vi "Experiment_Control.vi"() -> ()   [LabVIEW 2014]
uses:
  Controls/ExperimentControlEnum.ctl
  Controls/DAQ Channel Array.ctl
  Controls/DAQ Card-Channel Settings.ctl
  Controls/DAQ Card Channel Array.ctl
  Controls/DAQ Channel Settings.ctl
  Controls/DAQ Card Settings.ctl
  Controls/DIOTypedef.ctl
  Controls/TimingControlArray.ctl
  Controls/TimingControl.ctl
  Controls/TimingControlChannel.ctl
  Controls/TimeIncrementCluster.ctl
  Controls/TimingPlot.ctl
  Controls/ExperimentControlCluster.ctl
  Controls/ShotQualityEnum.ctl
panel:
  in  "Exit Program":bool
  in  "Restore Default Settings":bool
  in  "Tab Control":T1(tab)
  out "Program Version":string
  in  "Resume from previous shot":bool
  out "Timing Plot":T2
  in  "Load Shot Settings":bool
  in  "Load a previous shot?":i32
  in  "Shot Quality":enum32{"-2", "-1", "1", "2", "3", "0"}(radio)=enum."0"
  in  "Select MDS+ Data Tree":string(combo)="proto_tree"
  in  "Discard shot data":bool
  in  "Save shot data":bool
  in  "Increments":T3
  in  "Timing Array":T4 {"Timing Sequence"."Dt" format="%_3p"; "Timing Sequence"."Time" format="%_3p"}
  in  "Shot Notes":string
  out "Time":string
  out "System State":T7=enum."FIRE: Trigger"
  in  "Abort":bool
  in  "Fire Experiment":bool
  out "System Message":string
  out "Next Shot #":i32
  in  "DAQ Channel Array":T8 {"Card Settings"."Start Time" format="%#_3p"; "Card Settings"."End Time" format="%#_3p"; "Card Settings"."Rate" format="%#_3p"}
  in  "DIO Cluster":T13
  # "Save the current shot?"
  # "Time [s]"
  # "Channel                                     Name                                                               Voltage Range                    Card Settings"
  # "Sampling Rate [1/s]"
  # "Start Time [s]"
  # "End Time [s]"
  # "On/Off      Channel                     Name"
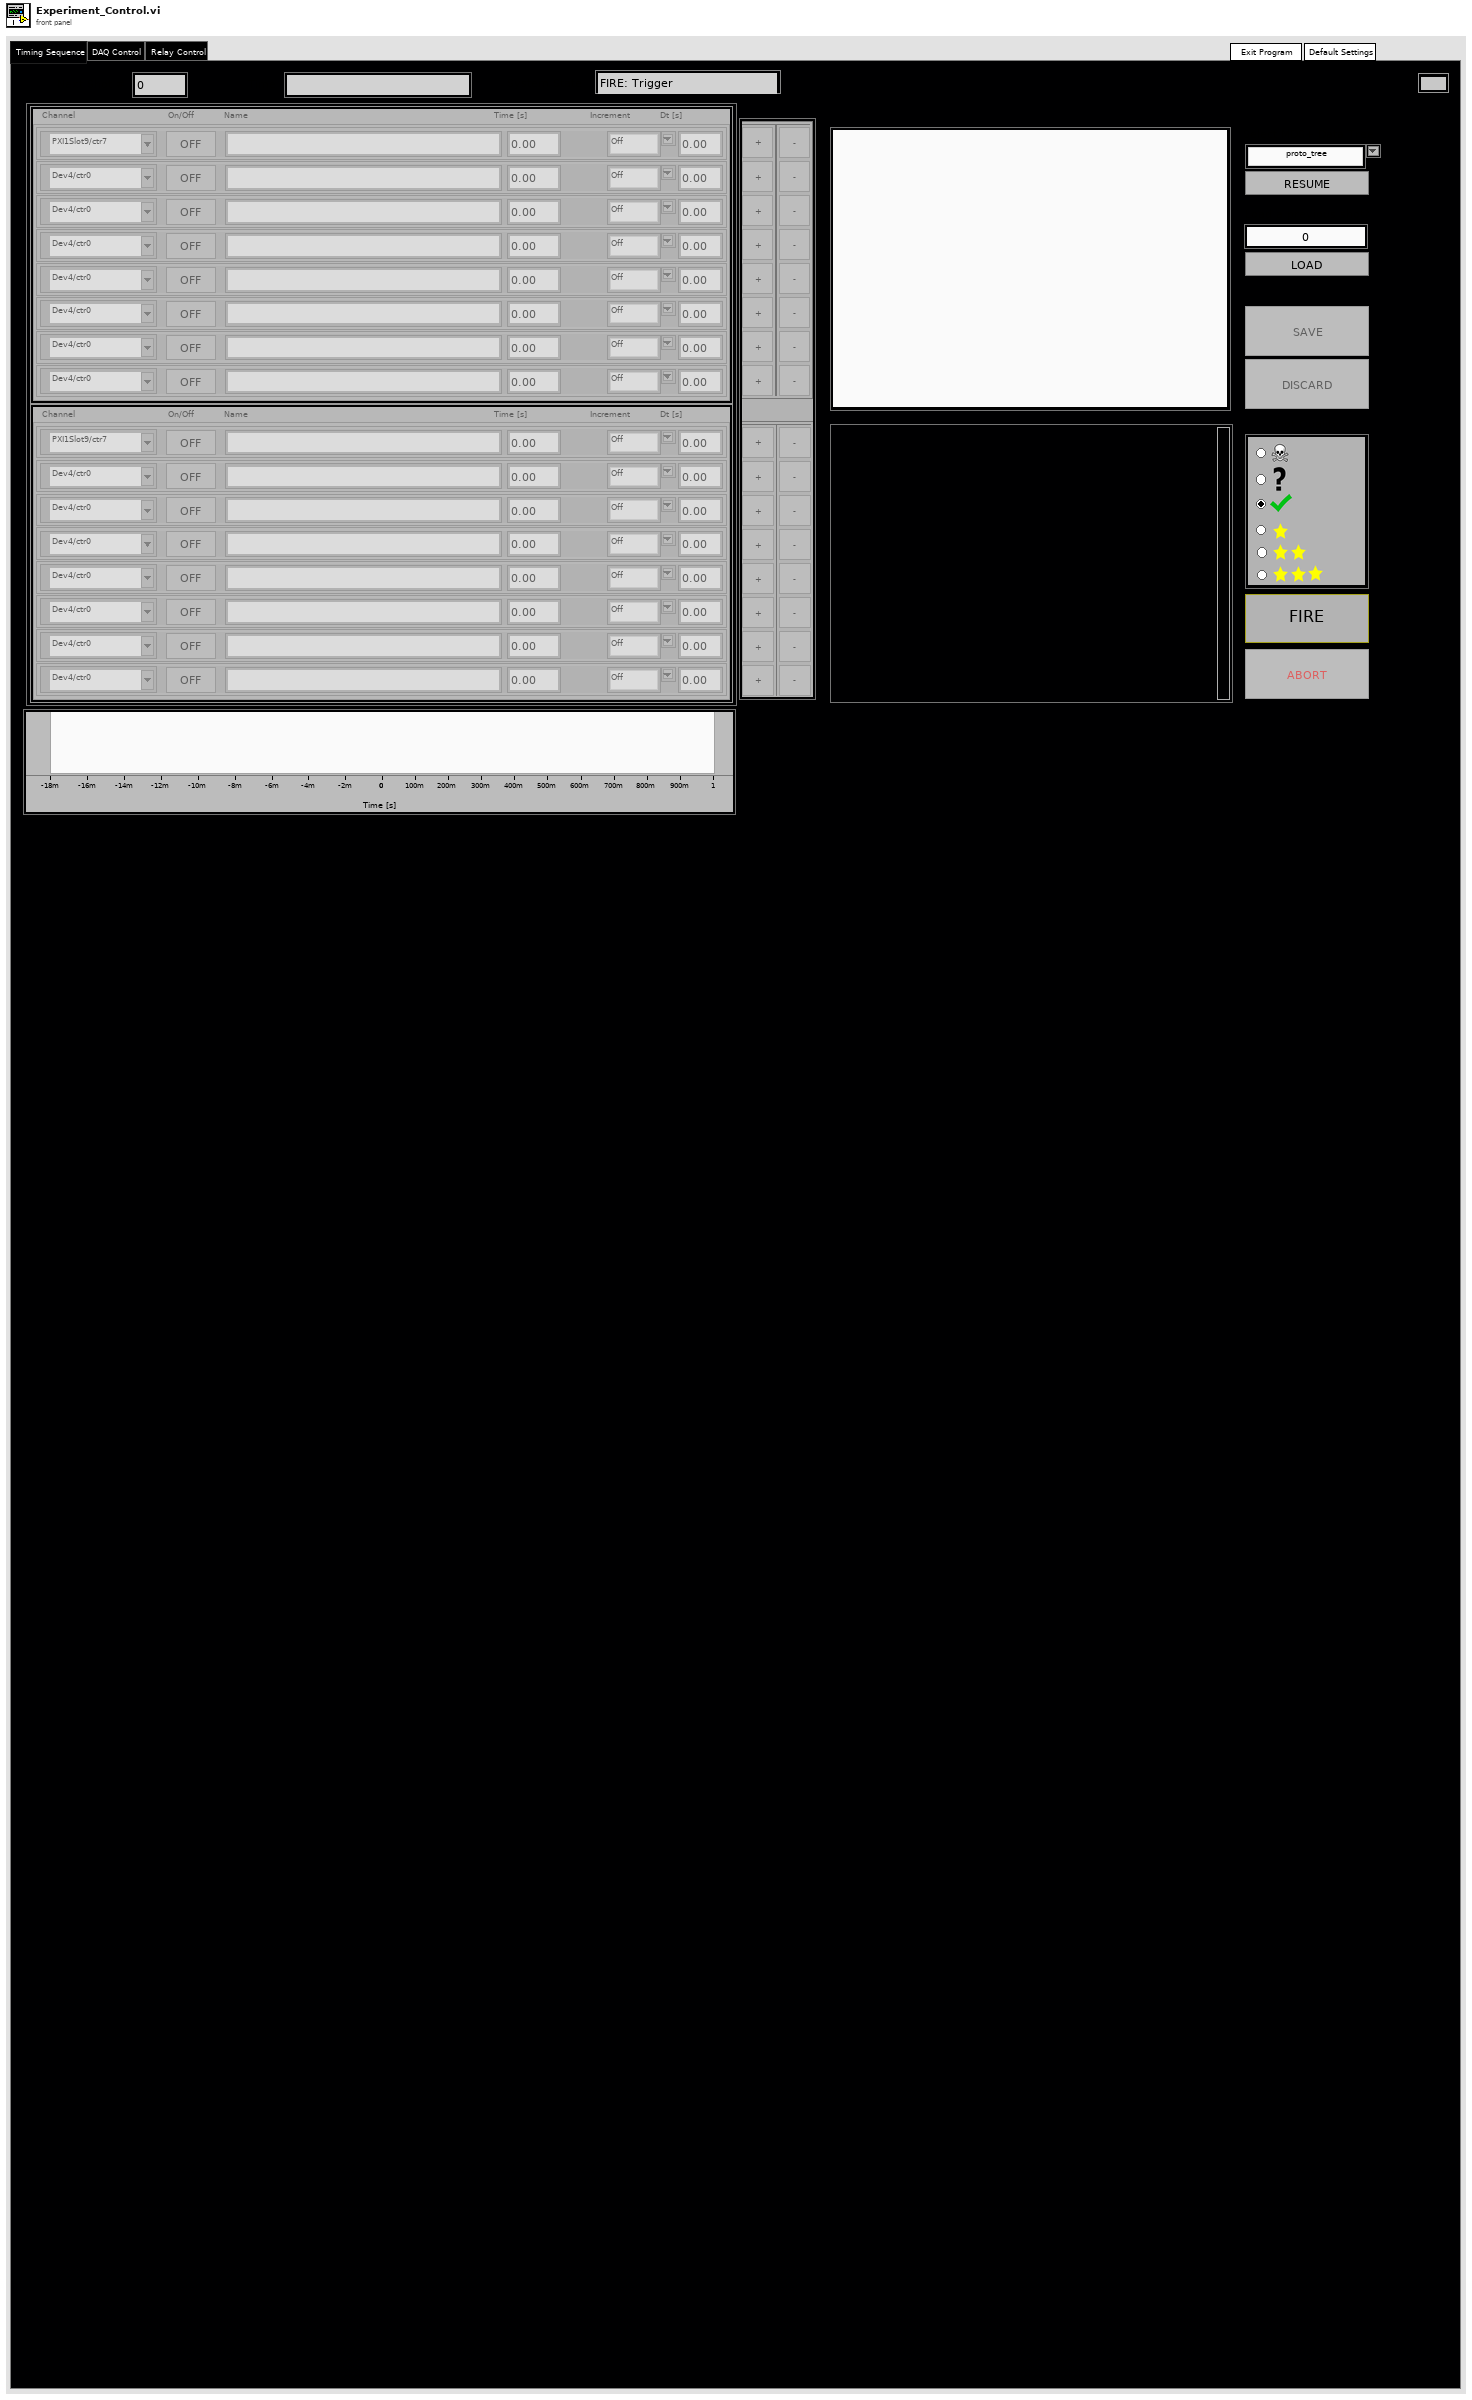
[diagram p1: front panel]
types:
  T1 = enum32{"Timing Sequence", "DAQ Control", "Relay Control"}
  T2 = typedef "TimingPlot.ctl" = cluster{"Negative Time Graph":cluster{dbl[], dbl[]}[], "Positive Time Graph":cluster{dbl[], dbl[]}[], "XY Graph":cluster{"X":dbl[], "Y":dbl[]}[]}
  T3 = typedef "TimeIncrementCluster.ctl" = cluster{"Plus Minus":cluster{"Add 1":cluster{"plus 1":bool, "plus 2":bool, "plus 3":bool, "plus 4":bool, "plus 5":bool, "plus 6":bool, "plus 7":bool, "plus 8":bool}, "Minus 1":cluster{"minus 1":bool, "minus 2":bool, "minus 3":bool, "minus 4":bool, "minus 5":bool, "minus 6":bool, "minus 7":bool, "minus 8":bool}}, "Plus Minus 2":cluster{"Add 1":cluster{"plus 1":bool, "plus 2":bool, "plus 3":bool, "plus 4":bool, "plus 5":bool, "plus 6":bool, "plus 7":bool, "plus 8":bool}, "Minus 1":cluster{"minus 1":bool, "minus 2":bool, "minus 3":bool, "minus 4":bool, "minus 5":bool, "minus 6":bool, "minus 7":bool, "minus 8":bool}}}
  T4 = typedef "TimingControlArray.ctl" = T5[]
  T5 = typedef "TimingControl.ctl" = cluster{"Timing Sequence":T6[]}
  T6 = typedef "TimingControlChannel.ctl" = cluster{"Active":bool, "counter":tag, "Channel Name":string, "Time":dbl, "Increment":string, "Dt":dbl}
  T7 = typedef "ExperimentControlEnum.ctl" = enum16{"Idle", "FIRE: Read Panel Settings", "FIRE: Generate Tasks", "FIRE: Set DAQ Triggers", "FIRE: Trigger", "FIRE: Wait for Task Completion", "FIRE: Read out DAQs", "Write to MDS+", "Clear Tasks", "Stop VI", "DIO Change", "Turn Off DIO", "Update Tree", "Load Shot Settings", "Restore Default Settings"}
  T8 = typedef "DAQ Channel Array.ctl" = T9[]
  T9 = typedef "DAQ Card-Channel Settings.ctl" = cluster{"DAQ Channel Array":T10, "Card Settings":T12}
  T10 = typedef "DAQ Card Channel Array.ctl" = T11[]
  T11 = typedef "DAQ Channel Settings.ctl" = cluster{"Active":bool, "Channel Name":string, "Channel":tag, "Voltage Range":string}
  T12 = typedef "DAQ Card Settings.ctl" = cluster{"Rate":dbl, "End Time":dbl, "Start Time":dbl}
  T13 = typedef "DIOTypedef.ctl" = cluster{"DIO Booleans":bool[], "DIO Channel Array":cluster{"Channel Name":string, "DIO lines":tag}[]}
  T14 = typedef "ExperimentControlCluster.ctl" = cluster{"Experiment Control":T7, "Variant":variant}
  T15 = typedef "ExperimentStateCluster.ctl" = cluster{"error":errorcluster, "Digitizer DAQmx Tasks":cluster{"TaskArray":refnum<k21>[]}, "Digitizer Settings":cluster{"Channel Settings":T16[][], "Card Settings":T17}, "Synchronization Settings":cluster{"Synchronizer":refnum<k15>, "source terminal":string}, "Digitizer Data":waveform(dbl)[][], "Next Shot#":string, "System Message":string, "User Shot Notes":string, "Timing Settings":T19, "Timing Tasks":cluster{"TaskArray":refnum<k21>[][]}, "Tree":string, "Time Card/Channels":i32[], "DAQ Card/Channels":i32[], "Program Version":string}
  T16 = typedef "DigitizerSettingsChannelSettings.ctl" = cluster{"Channel":tag, "Channel Name":string, "Voltage Range":dbl, "Active":bool}
  T17 = typedef "DigitizerSettingsCardSettingsArray.ctl" = T18[]
  T18 = typedef "DigitizerSettingsCardSettings.ctl" = cluster{"Start Time":dbl, "End Time":dbl, "Sample Rate":dbl, " Pre-Trigger Samples":u32, "Total Samples":i32, "Samples to Remove":u32, "Trigger Source":tag, "Global Edge Type":i32, "PXIStarLine":tag}
  T19 = typedef "TimingSettings.ctl" = cluster{"Timing Card Settings":T20[], "Timing Channel Settings":T21[][]}
  T20 = typedef "TimingCardSettings.ctl" = cluster{"Trigger Source":tag, "Clock Source":tag, "PXIStarLine":tag}
  T21 = typedef "TimingChannelSettings.ctl" = cluster{"Delay (s)":dbl, "Pulse width (s)":dbl, "Active":bool, "Channel Name":string, "counter":tag, "FrontPanelTime":dbl}
  T22 = cluster{"DAQ Channel Array":T10, "Card Settings":T12}[]
  T23 = typedef "ShotQualityEnum.ctl" = enum32{"-2", "-1", "1", "2", "3", "0"}
  T24 = cluster{"Channel Name":string, "DIO lines":tag}[]
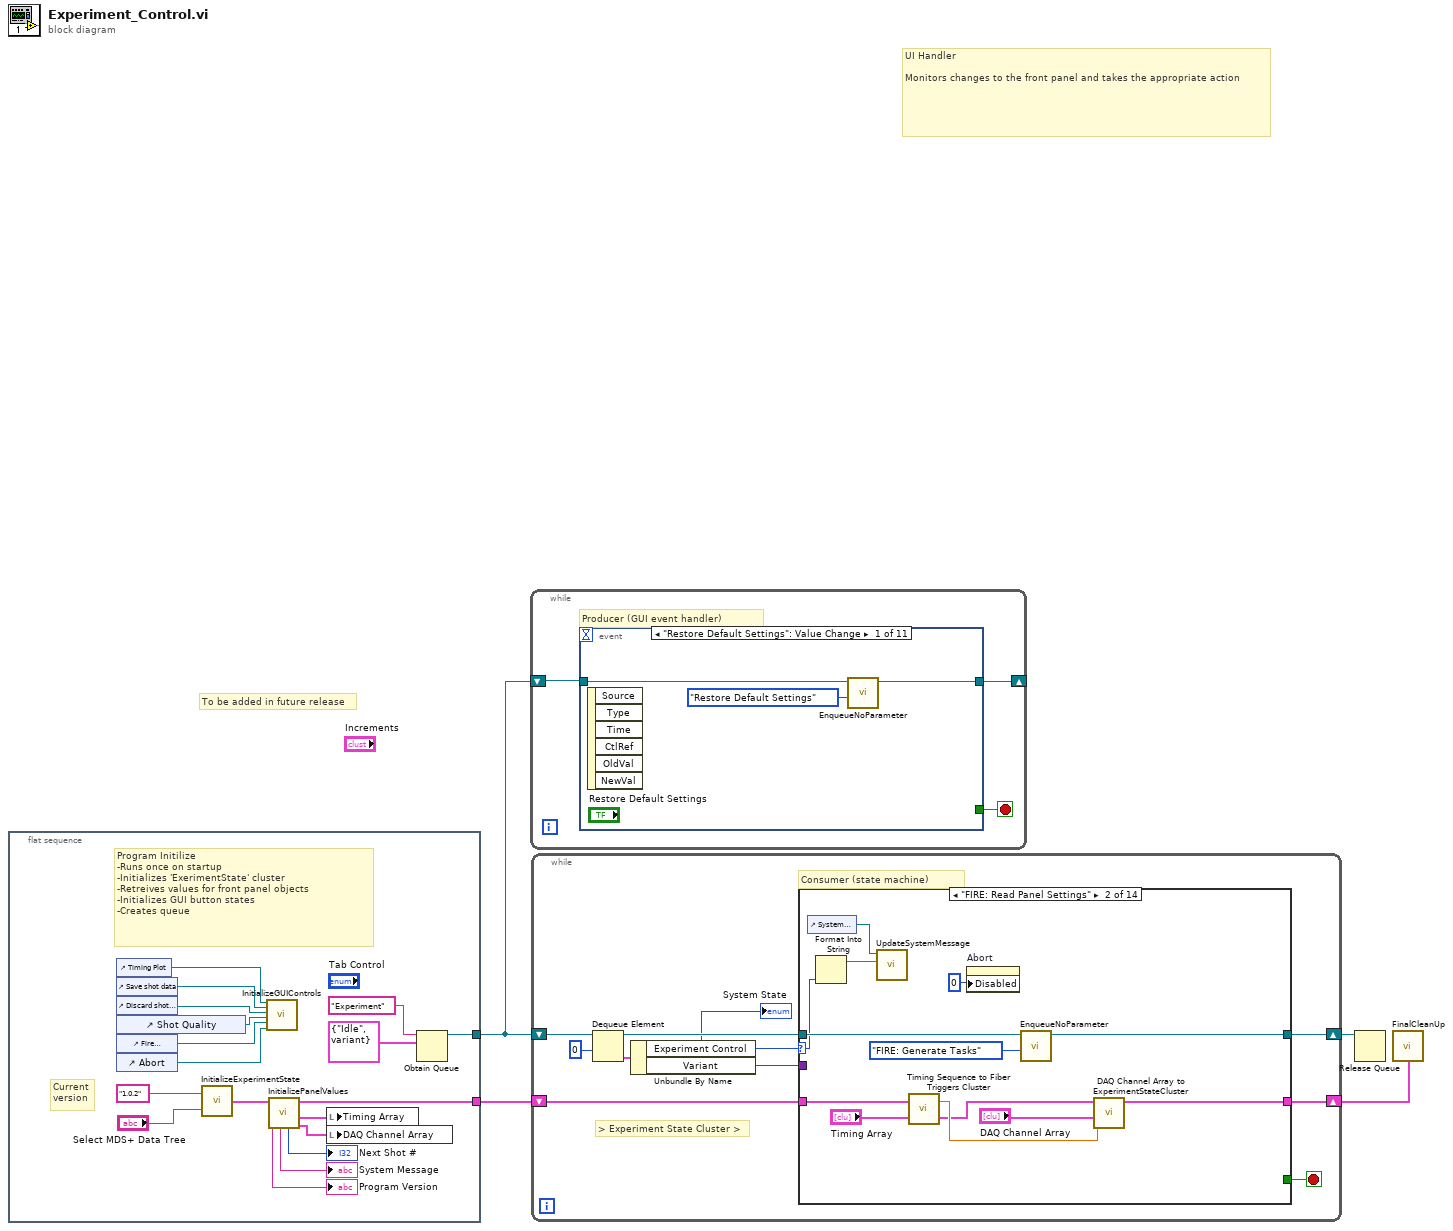
[diagram p0: block diagram]
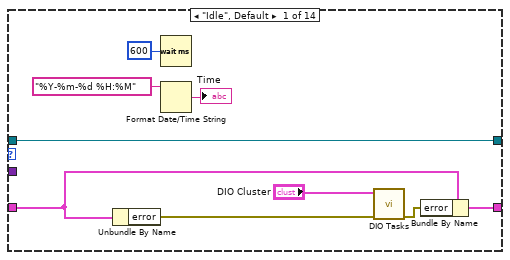
[diagram p2: hidden frame]
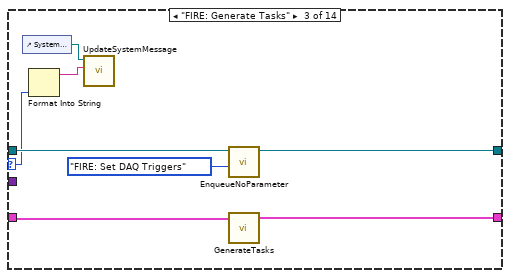
[diagram p3: hidden frame]
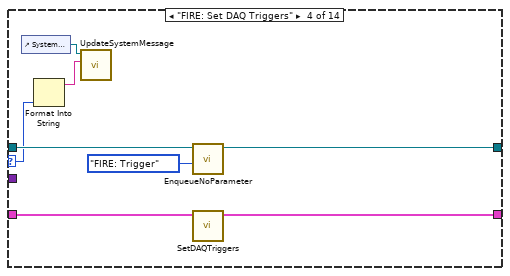
[diagram p4: hidden frame]
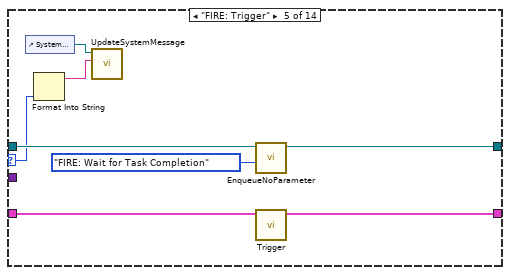
[diagram p5: hidden frame]
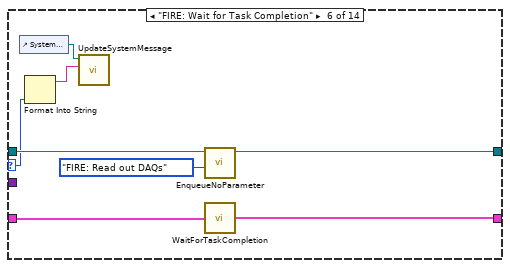
[diagram p6: hidden frame]
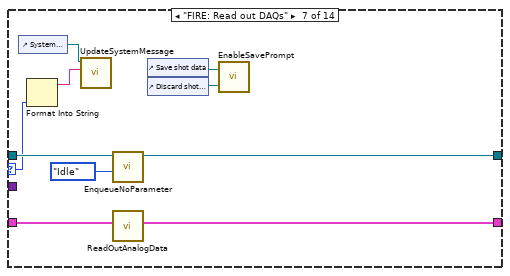
[diagram p7: hidden frame]
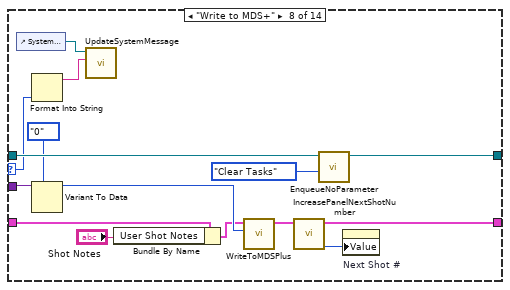
[diagram p8: hidden frame]
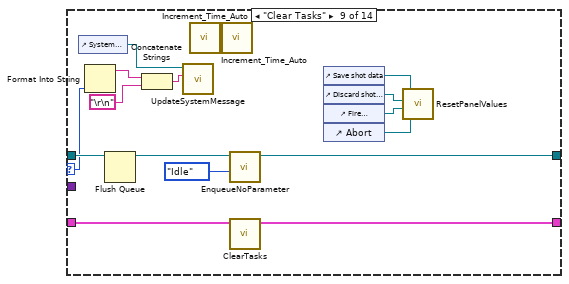
[diagram p9: hidden frame]
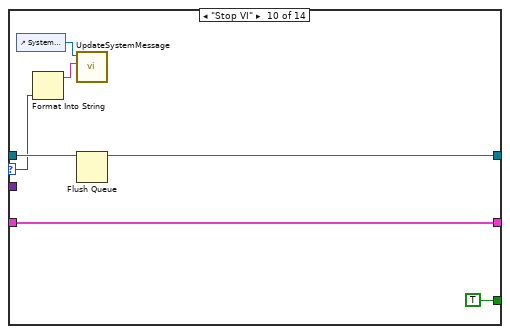
[diagram p10: hidden frame]
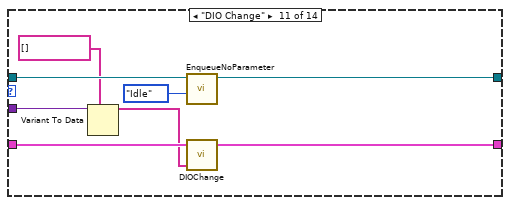
[diagram p11: hidden frame]
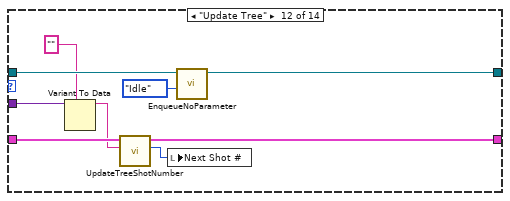
[diagram p12: hidden frame]
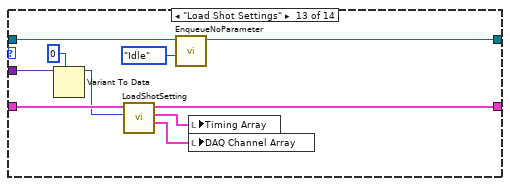
[diagram p13: hidden frame]
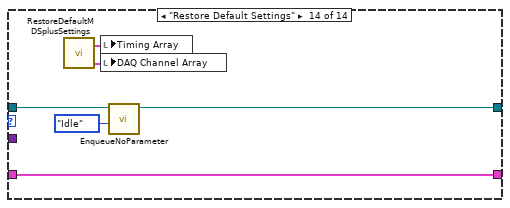
[diagram p14: hidden frame]
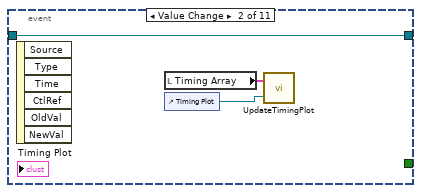
[diagram p15: hidden frame]
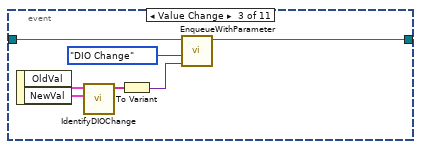
[diagram p16: hidden frame]
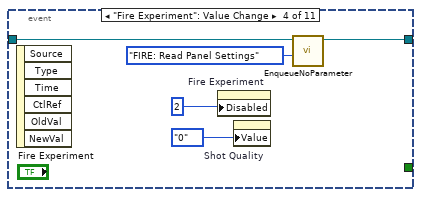
[diagram p17: hidden frame]
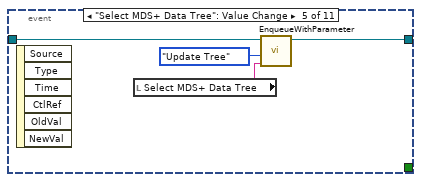
[diagram p18: hidden frame]
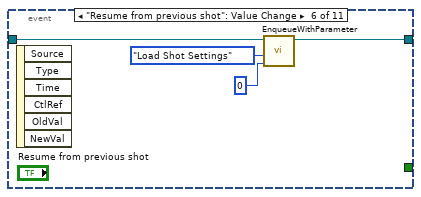
[diagram p19: hidden frame]
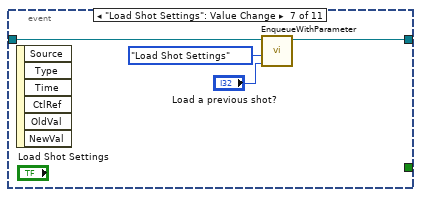
[diagram p20: hidden frame]
diagram:
  # "To be added in future release"
  # "UI Handler\n\nMonitors changes to the front panel and takes the appropriate action"
  n1 = flat-sequence {
    tunnel: [w21] -> w4
    tunnel: [w10] -> w3
    frame #0 {
      # "Current\nversion"
      # "Program Initilize\n-Runs once on startup\n-Initializes 'ExerimentState' cluster\n-Retreives values for front panel objects\n-Initializes GUI button states\n-Creates queue"
      n2 = control-ref of="Timing Plot"() -> (w17:refnum<vi>)
      n3 = control-ref of="Save shot data"() -> (w16:refnum<vi>)
      n4 = control-ref of="Discard shot data"() -> (w15:refnum<vi>)
      n5 = control-ref of="Shot Quality"() -> (w12:refnum<vi>)
      n6 = control-ref of="Fire Experiment"() -> (w13:refnum<vi>)
      n7 = control-ref of="Abort"() -> (w14:refnum<vi>)
      n8 = call "InitializeExperimentState.vi"("Tree Name"="Select MDS+ Data Tree", "Program Version"="1.0.2" ("string")) -> ("Experiment State"=w11:T15)
      n9 = call "InitializeGUIControls.vi"("Timing Plot"=w17, "Save shot data"=w16, "Discard shot data"=w15, "Shot Quality"=w12, "Fire Experiment"=w13, "Abort"=w14) -> ()  [unwired: 14 in]
      n10 = call "InitializePanelValues.vi"("Experiment State in"=w11) -> ("Initialized DAQ Array"=w8:T22, "Initialized Timing Array"=w9:T5[], "Experiment State out"=w10:T15, "Next Shot #"=→"Next Shot #":i32, "System Message"=→"System Message":string, "Program Version"=→"Program Version":string)  [unwired: 5 in]
      n11 = local write "Timing Array"(w9) -> ()
      n12 = local write "DAQ Channel Array"(w8) -> ()
      n13 = Obtain Queue(name (unnamed)="Experiment", element data type=T14 {"Experiment Control"=enum."Idle", "Variant"=variant} ("ExperimentControl")) -> (queue out=w21:refnum<queue>)  [unwired: 3 in, 2 out]
    }
  }
  n14 = while {
    shift-right: [w23] -> _
    shift-left: w4 -> [w25]
    stop <- w24 stop-if-true
    # "Producer (GUI event handler)"
    n15 = event shown="[0] \"Restore Default Settings\": Value Change" {
      selector: _ -> [_ _ _ _ _ _ _ _ _ _ _]
      dyn-events: _ -> [_ _ _ _ _ _ _ _ _ _ _]
      timeout: _ -> [_ _ _ _ _ _ _ _ _ _ _]
      tunnel: w25 -> [w28 w31 w35 w43 w47 w50 w55 w60 w63 w66 w69]
      tunnel: [w27 w31 w36 w42 w46 w49 w54 w59 w62 w65 w68] -> w23
      tunnel: [_ _ _ _ _ _ _ _ _ _ TRUE] -> w24
      event "Restore Default Settings": Value Change {
        n16 = event-data() -> ()  [unwired: 7 out]
        n17 = call "EnqueueNoParameter.vi"("Command"=ExperimentControlEnum."Restore Default Settings", "Command Q"=w28) -> ("Command Q"=w27:refnum<queue>)  [unwired: 9 in]
      }
      event Value Change {
        n18 = event-data() -> ()  [unwired: 7 out]
        n19 = local read "Timing Array"() -> (w29:T4)
        n20 = control-ref of="Timing Plot"() -> (w30:refnum<vi>)
        n21 = call "UpdateTimingPlot.vi"("Ctl Refnum"=w30, "TimingArray"=w29) -> ()  [unwired: 2 in]
      }
      event Value Change {
        n22 = event-data() -> ("OldVal"=w38:T24, "NewVal"=w37:T24)  [unwired: 1 out]
        n23 = call "IdentifyDIOChange.vi"("NewVal"=w37, "OldVal"=w38) -> ("Changed DIO"=w33:tag[])  [unwired: 9 in]
        n24 = To Variant(anything=w33) -> (Variant=w32:variant)
        n25 = call "EnqueueWithParameter.vi"("Parameter"=w32, "Command"=ExperimentControlEnum."DIO Change", "Command Q"=w35) -> ("Command Q"=w36:refnum<queue>)  [unwired: 8 in]
      }
      event "Fire Experiment": Value Change {
        n26 = event-data() -> ()  [unwired: 7 out]
        n27 = property on="Fire Experiment" class="Bool"("Disabled"=u8 2) -> ()  [unwired: 2 in, 2 out]
        n28 = property on="Shot Quality" class="RadioBtnsControl (strict)"("Value"=ShotQualityEnum."0" ("Shot Quality")) -> ()  [unwired: 2 in, 2 out]
        n29 = call "EnqueueNoParameter.vi"("Command"=ExperimentControlEnum."FIRE: Read Panel Settings", "Command Q"=w43) -> ("Command Q"=w42:refnum<queue>)  [unwired: 9 out]
      }
      event "Select MDS+ Data Tree": Value Change {
        n30 = event-data() -> ()  [unwired: 7 out]
        n31 = local read "Select MDS+ Data Tree"() -> (w44:string)
        n32 = call "EnqueueWithParameter.vi"("Parameter"=w44, "Command"=ExperimentControlEnum."Update Tree", "Command Q"=w47) -> ("Command Q"=w46:refnum<queue>)  [unwired: 8 in]
      }
      event "Resume from previous shot": Value Change {
        n33 = event-data() -> ()  [unwired: 7 out]
        n34 = call "EnqueueWithParameter.vi"("Parameter"=0, "Command"=ExperimentControlEnum."Load Shot Settings", "Command Q"=w50) -> ("Command Q"=w49:refnum<queue>)  [unwired: 8 in]
      }
      event "Load Shot Settings": Value Change {
        n35 = event-data() -> ()  [unwired: 7 out]
        n36 = call "EnqueueWithParameter.vi"("Parameter"="Load a previous shot?", "Command"=ExperimentControlEnum."Load Shot Settings", "Command Q"=w55) -> ("Command Q"=w54:refnum<queue>)  [unwired: 8 in]
      }
      event "Save shot data": Value Change {
        n37 = event-data() -> ()  [unwired: 7 out]
        n38 = To Variant(anything="Shot Quality") -> (Variant=w58:variant)
        n39 = call "EnqueueWithParameter.vi"("Parameter"=w58, "Command"=ExperimentControlEnum."Write to MDS+", "Command Q"=w60) -> ("Command Q"=w59:refnum<queue>)  [unwired: 8 in]
      }
      event "Discard shot data": Value Change {
        n40 = event-data() -> ()  [unwired: 7 out]
        n41 = call "EnqueueNoParameter.vi"("Command"=ExperimentControlEnum."Clear Tasks", "Command Q"=w63) -> ("Command Q"=w62:refnum<queue>)  [unwired: 9 out]
      }
      event "Abort": Value Change {
        n42 = event-data() -> ()  [unwired: 7 out]
        n43 = call "EnqueueNoParameter.vi"("Command"=ExperimentControlEnum."Clear Tasks", "Command Q"=w66) -> ("Command Q"=w65:refnum<queue>)  [unwired: 9 out]
      }
      event "Exit Program": Value Change {
        n44 = event-data() -> ()  [unwired: 7 out]
        n45 = call "EnqueueNoParameter.vi"("Command"=ExperimentControlEnum."Stop VI", "Command Q"=w69) -> ("Command Q"=w68:refnum<queue>)  [unwired: 9 in]
      }
    }
  }
  n46 = while {
    shift-right: [w79] -> w1
    shift-left: w4 -> [w80]
    shift-right: [w75] -> w2
    shift-left: w3 -> [w74]
    stop <- w73 stop-if-true
    # "Consumer (state machine)"
    # "> Experiment State Cluster >"
    n47 = Dequeue Element(queue=w80, timeout in ms (-1)=0) -> (queue out=w78:refnum<queue>, element=w76:T14)  [unwired: 1 in, 2 out]
    n48 = Unbundle By Name(w76) -> ("Experiment Control"=w72:T7, "Variant"=w71:variant)
    "System State" <- w72
    n49 = case shown="\"FIRE: Read Panel Settings\"" w72 {
      selector: w72 -> [_ w91 w105 w114 w122 w129 w140 w156 w169 w177 _ _ _ _]
      tunnel: [w89 w101 w106 w116 w123 w132 w141 w157 w171 w178 w188 w197 w207 w213] -> w79
      tunnel: w78 -> [w89 w102 w107 w117 w124 w133 w142 w158 w174 w179 w189 w198 w208 w214]
      tunnel: [w81 w98 w109 w115 w119 w130 w139 w155 w160 w181 w185 w194 w203 w212] -> w75
      tunnel: w74 -> [w82 w94 w110 w111 w126 w131 w144 w152 w170 w181 w186 w191 w200 w212]
      tunnel: [_ _ _ _ _ _ _ _ _ TRUE _ _ _ _] -> w73
      tunnel: w71 -> [_ _ _ _ _ _ _ w153 _ _ w184 w193 w205 _]
      frame "Idle", Default {
        n50 = Unbundle By Name(w82) -> ("error"=w84:errorcluster)
        n51 = Wait (ms)(milliseconds to wait=u32 600 ("millisecond multiple")) -> ()  [unwired: 1 out]
        n52 = Format Date/Time String(time format string (%c)="%Y-%m-%d %H:%M") -> (date/time string=→"Time":string)  [unwired: 2 in]
        n53 = call "DIO Tasks.vi"("error in"=w84, "DIO Cluster"="DIO Cluster") -> ("error out"=w83:errorcluster)  [unwired: 9 in]
        n54 = Bundle By Name(cluster=w82, "error"=w83) -> (w81:T15)
      }
      frame "FIRE: Read Panel Settings" {
        n55 = control-ref of="System Message"() -> (w92:refnum<vi>)
        n56 = Format Into String(w91) -> (resulting string=w90:string)  [unwired: 3 in, 1 out]
        n57 = call "UpdateSystemMessage.vi"("Message"=w90, "System Message Terminal Ref In"=w92) -> ()  [unwired: 10 in]
        n58 = call "Timing Sequence to Fiber Triggers Cluster.vi"("Timing Control Array"="Timing Array", "Experiment State In"=w94) -> ("Experiment State Out"=w93:T15, "First trigger time"=w97:dbl)
        n59 = property on="Abort" class="Bool (strict)"("Disabled"=u8 0) -> ()  [unwired: 2 in, 2 out]
        n60 = call "EnqueueNoParameter.vi"("Command"=ExperimentControlEnum."FIRE: Generate Tasks" ("Experiment Control"), "Command Q"=w102) -> ("Command Q"=w101:refnum<queue>)  [unwired: 9 out]
        n61 = call "DAQ Channel Array to ExperimentStateCluster.vi"("First Trigger Time"=w97, "DAQ Channel Array"="DAQ Channel Array", "Experiment State"=w93) -> ("Experiment State Out"=w98:T15)  [unwired: 8 in]
      }
      frame "FIRE: Generate Tasks" {
        n62 = control-ref of="System Message"() -> (w104:refnum<vi>)
        n63 = Format Into String(w105) -> (resulting string=w103:string)  [unwired: 3 in, 1 out]
        n64 = call "UpdateSystemMessage.vi"("Message"=w103, "System Message Terminal Ref In"=w104) -> ()  [unwired: 10 in]
        n65 = call "EnqueueNoParameter.vi"("Command"=ExperimentControlEnum."FIRE: Set DAQ Triggers" ("Experiment Control"), "Command Q"=w107) -> ("Command Q"=w106:refnum<queue>)  [unwired: 9 out]
        n66 = call "GenerateTasks.vi"("Experiment State"=w110) -> ("Experiment State"=w109:T15)  [unwired: 1 in, 9 out]
      }
      frame "FIRE: Set DAQ Triggers" {
        n67 = control-ref of="System Message"() -> (w112:refnum<vi>)
        n68 = Format Into String(w114) -> (resulting string=w113:string)  [unwired: 3 in, 1 out]
        n69 = call "UpdateSystemMessage.vi"("Message"=w113, "System Message Terminal Ref In"=w112) -> ()  [unwired: 10 in]
        n70 = call "EnqueueNoParameter.vi"("Command"=ExperimentControlEnum."FIRE: Trigger" ("Experiment Control"), "Command Q"=w117) -> ("Command Q"=w116:refnum<queue>)  [unwired: 9 out]
        n71 = call "SetDAQTriggers.vi"("Experiment State in"=w111) -> ("Experiment State out 2"=w115:T15)  [unwired: 10 in]
      }
      frame "FIRE: Trigger" {
        n72 = control-ref of="System Message"() -> (w121:refnum<vi>)
        n73 = Format Into String(w122) -> (resulting string=w120:string)  [unwired: 3 in, 1 out]
        n74 = call "UpdateSystemMessage.vi"("Message"=w120, "System Message Terminal Ref In"=w121) -> ()  [unwired: 10 in]
        n75 = call "EnqueueNoParameter.vi"("Command"=ExperimentControlEnum."FIRE: Wait for Task Completion" ("Experiment Control"), "Command Q"=w124) -> ("Command Q"=w123:refnum<queue>)  [unwired: 9 out]
        n76 = call "Trigger.vi"("Experiment State in"=w126) -> ("Experiment State Out"=w119:T15)  [unwired: 10 in]
      }
      frame "FIRE: Wait for Task Completion" {
        n77 = control-ref of="System Message"() -> (w127:refnum<vi>)
        n78 = Format Into String(w129) -> (resulting string=w128:string)  [unwired: 3 in, 1 out]
        n79 = call "UpdateSystemMessage.vi"("Message"=w128, "System Message Terminal Ref In"=w127) -> ()  [unwired: 10 in]
        n80 = call "EnqueueNoParameter.vi"("Command"=ExperimentControlEnum."FIRE: Read out DAQs" ("Experiment Control"), "Command Q"=w133) -> ("Command Q"=w132:refnum<queue>)  [unwired: 9 out]
        n81 = call "WaitForTaskCompletion.vi"("Experiment State"=w131) -> ("Experiment State"=w130:T15)  [unwired: 10 out]
      }
      frame "FIRE: Read out DAQs" {
        n82 = control-ref of="System Message"() -> (w137:refnum<vi>)
        n83 = Format Into String(w140) -> (resulting string=w138:string)  [unwired: 3 in, 1 out]
        n84 = call "UpdateSystemMessage.vi"("Message"=w138, "System Message Terminal Ref In"=w137) -> ()  [unwired: 10 in]
        n85 = call "EnqueueNoParameter.vi"("Command"=ExperimentControlEnum."Idle" ("Experiment Control"), "Command Q"=w142) -> ("Command Q"=w141:refnum<queue>)  [unwired: 9 out]
        n86 = call "ReadOutAnalogData.vi"("Experiment State"=w144) -> ("Experiment State"=w139:T15)  [unwired: 10 out]
        n87 = control-ref of="Save shot data"() -> (w136:refnum<vi>)
        n88 = control-ref of="Discard shot data"() -> (w135:refnum<vi>)
        n89 = call "EnableSavePrompt.vi"("Discard shot data"=w135, "Save shot data"=w136) -> ()  [unwired: 2 in]
      }
      frame "Write to MDS+" {
        n90 = control-ref of="System Message"() -> (w148:refnum<vi>)
        n91 = Format Into String(w156) -> (resulting string=w149:string)  [unwired: 3 in, 1 out]
        n92 = Variant To Data(type=ShotQualityEnum."0" ("Shot Quality"), Variant=w153) -> (data=w151:T23)  [unwired: 1 in, 1 out]
        n93 = call "UpdateSystemMessage.vi"("Message"=w149, "System Message Terminal Ref In"=w148) -> ()  [unwired: 10 in]
        n94 = Bundle By Name(cluster=w152, "User Shot Notes"="Shot Notes") -> (w147:T15)
        n95 = call "WriteToMDSPlus.vi"("Shot Quality"=w151, "Experiment State in"=w147) -> ("Experiment State out"=w146:T15)  [unwired: 9 in]
        n96 = call "IncreasePanelNextShotNumber.vi"("Experiment State in"=w146) -> ("Next shot #"=w145:i32, "Experiment State out"=w155:T15)  [unwired: 9 in]
        n97 = call "EnqueueNoParameter.vi"("Command"=ExperimentControlEnum."Clear Tasks" ("Experiment Control"), "Command Q"=w158) -> ("Command Q"=w157:refnum<queue>)  [unwired: 9 out]
        n98 = property on="Next Shot #" class="DigNum (strict)"("Value"=w145) -> ()  [unwired: 2 in, 2 out]
      }
      frame "Clear Tasks" {
        n99 = control-ref of="System Message"() -> (w168:refnum<vi>)
        n100 = Format Into String(w169) -> (resulting string=w165:string)  [unwired: 3 in, 1 out]
        n101 = Flush Queue(queue=w174) -> (queue out=w172:refnum<queue>)  [unwired: 1 in, 2 out]
        n102 = Concatenate Strings(w165, "\r\n") -> (w167:string)
        n103 = call "UpdateSystemMessage.vi"("Message"=w167, "System Message Terminal Ref In"=w168) -> ()  [unwired: 10 in]
        n104 = call "Increment_Time_Auto.vi"() -> ()  [unwired: 11 in, 1 out]
        n105 = call "Increment_Time_Auto.vi"() -> ()  [unwired: 11 in, 1 out]
        n106 = call "EnqueueNoParameter.vi"("Command"=ExperimentControlEnum."Idle" ("Experiment Control"), "Command Q"=w172) -> ("Command Q"=w171:refnum<queue>)  [unwired: 9 out]
        n107 = call "ClearTasks.vi"("Experiment State in"=w170) -> ("Experiment State out"=w160:T15)  [unwired: 10 in]
        n108 = control-ref of="Save shot data"() -> (w164:refnum<vi>)
        n109 = control-ref of="Discard shot data"() -> (w163:refnum<vi>)
        n110 = control-ref of="Fire Experiment"() -> (w162:refnum<vi>)
        n111 = control-ref of="Abort"() -> (w161:refnum<vi>)
        n112 = call "ResetPanelValues.vi"("Abort"=w161, "Fire Experiment"=w162, "Discard shot data"=w163, "Save shot data"=w164) -> ()  [unwired: 4 in]
      }
      frame "Stop VI" {
        n113 = control-ref of="System Message"() -> (w176:refnum<vi>)
        n114 = Format Into String(w177) -> (resulting string=w175:string)  [unwired: 3 in, 1 out]
        n115 = call "UpdateSystemMessage.vi"("Message"=w175, "System Message Terminal Ref In"=w176) -> ()  [unwired: 10 in]
        n116 = Flush Queue(queue=w179) -> (queue out=w178:refnum<queue>)  [unwired: 1 in, 2 out]
      }
      frame "DIO Change" {
        n117 = Variant To Data(type=tag[] [] ("Changed DIO"), Variant=w184) -> (data=w182:tag[])  [unwired: 1 in, 1 out]
        n118 = call "EnqueueNoParameter.vi"("Command"=ExperimentControlEnum."Idle", "Command Q"=w189) -> ("Command Q"=w188:refnum<queue>)  [unwired: 9 out]
        n119 = call "DIOChange.vi"("Changed DIO"=w182, "Experiment State in"=w186) -> ("Experiment State out"=w185:T15)  [unwired: 3 in]
      }
      frame "Update Tree" {
        n120 = Variant To Data(type="", Variant=w193) -> (data=w190:string)  [unwired: 1 in, 1 out]
        n121 = call "UpdateTreeShotNumber.vi"("Tree name"=w190, "Experiment State in"=w191) -> ("Numeric"=w195:i32, "Experiment State out"=w194:T15)  [unwired: 8 in]
        n122 = local write "Next Shot #"(w195) -> ()
        n123 = call "EnqueueNoParameter.vi"("Command"=ExperimentControlEnum."Idle", "Command Q"=w198) -> ("Command Q"=w197:refnum<queue>)  [unwired: 9 in]
      }
      frame "Load Shot Settings" {
        n124 = Variant To Data(type=0, Variant=w205) -> (data=w199:i32)  [unwired: 1 in, 1 out]
        n125 = call "LoadShotSetting.vi"("Shot Number"=w199, "Experiment State in"=w200) -> ("Initialized DAQ Array"=w201:T22, "Initialized Timing Array"=w202:T5[], "Experiment State OUT"=w203:T15)  [unwired: 7 in]
        n126 = call "EnqueueNoParameter.vi"("Command"=ExperimentControlEnum."Idle", "Command Q"=w208) -> ("Command Q"=w207:refnum<queue>)  [unwired: 9 in]
        n127 = local write "Timing Array"(w202) -> ()
        n128 = local write "DAQ Channel Array"(w201) -> ()
      }
      frame "Restore Default Settings" {
        n129 = call "RestoreDefaultMDSplusSettings.vi"() -> ("Initialized DAQ Array"=w209:T22, "Initialized Timing Array"=w210:T5[])  [unwired: 2 in]
        n130 = local write "Timing Array"(w210) -> ()
        n131 = local write "DAQ Channel Array"(w209) -> ()
        n132 = call "EnqueueNoParameter.vi"("Command"=ExperimentControlEnum."Idle", "Command Q"=w214) -> ("Command Q"=w213:refnum<queue>)  [unwired: 9 out]
      }
    }
  }
  n133 = Release Queue(queue=w1) -> ()  [unwired: 2 in, 3 out]
  n134 = call "FinalCleanUp.vi"("Experiment State in"=w2) -> ()
